vi "ParseInputs.vi"(8 "error in (no error)":errorcluster, 10 "Inputs":string[](array[string]), 11 "DiscoverTestCases in":refnum<class "DiscoverTestCases.lvclass">) -> (0 "error out":errorcluster, 3 "DiscoverTestCases out":refnum<class "DiscoverTestCases.lvclass">)   [LabVIEW 2015, in "DiscoverTestCases.lvclass"]
uses:
  DiscoverTestCases.lvclass
  DiscoverTestCases.lvclass/DiscoverTestCases.ctl
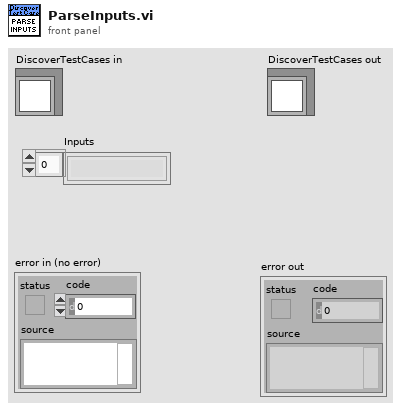
[diagram p1: front panel]
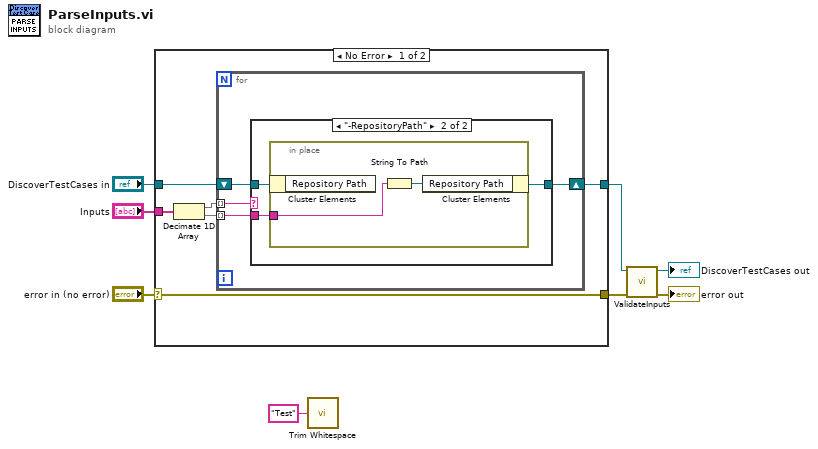
[diagram p0: block diagram]
diagram:
  n1 = case shown="No Error" "error in (no error)" {
    selector: "error in (no error)" -> [w9 w26]
    tunnel: [w9 w26] -> w3
    tunnel: "Inputs" -> [w14 _]
    tunnel: "DiscoverTestCases in" -> [w11 w25]
    tunnel: [w10 w25] -> w5
    frame No Error {
      n2 = Decimate 1D Array(w14) -> (w13:string[], w12:string[])
      n3 = for {
        tunnel: w13 -> [w18] mode=indexing
        tunnel: w12 -> [w15] mode=indexing
        shift-right: [w16] -> w10
        shift-left: w11 -> [w17]
        n4 = case shown="\"-RepositoryPath\"" w18 {
          tunnel: w17 -> [w19 w22]
          tunnel: [w19 w21] -> w16
          tunnel: w15 -> [_ w20]
          frame Default {
          }
          frame "-RepositoryPath" {
            n5 = in-place {
              in-place-border: w20 -> [w23]
              n6 = in-place-cluster #1(w22) -> ()  [unwired: 1 out]
              n7 = String To Path(string=w23) -> (path=w24:path)
              n8 = in-place-cluster #1("Repository Path"=w24) -> (w21:refnum<class "DiscoverTestCases.lvclass">)
            }
          }
        }
      }
    }
    frame Error {
    }
  }
  n9 = call <vilib>:"Trim Whitespace.vi"("string"="Test") -> ()  [unwired: 1 in, 1 out]
  n10 = call "ValidateInputs.vi"("error in (no error)"=w3, "DiscoverTestCases in"=w5) -> ("error out"=→"error out":errorcluster, "DiscoverTestCases out"=→"DiscoverTestCases out":refnum<class "DiscoverTestCases.lvclass">)  [unwired: 8 in]
